vi "Send Example.vi"(0 "Input Data":T1 {"Command" format="%02x"; "Destination" format="%02x"; "Source" format="%02x"}, 1 "Retry Count":u8=5, 5 "Timeout (ms)":u32=500, 7 "Wait for Acknowledgement?":bool, 11 "Error In":errorcluster) -> (15 "Error Out":errorcluster)   [LabVIEW 2016]
doc: "This standalone VI sends a GEA2 message to the destination you specify."
uses:
  LabVIEW_GEA2_Toolkit.lvlibp/type defs/Data In.ctl
  LabVIEW_GEA2_Toolkit.lvlibp
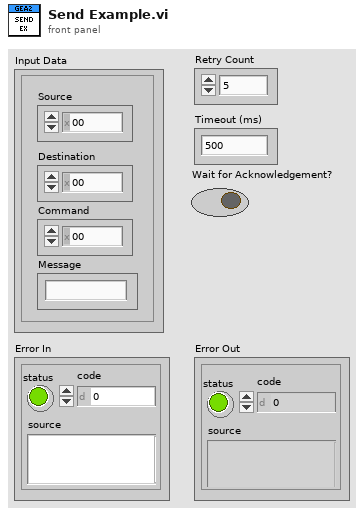
[diagram p1: front panel]
types:
  T1 = typedef "LabVIEW_GEA2_Toolkit.lvlibp/Data In.ctl" = cluster{"Source":u8, "Destination":u8, "Command":u8, "Message":string}
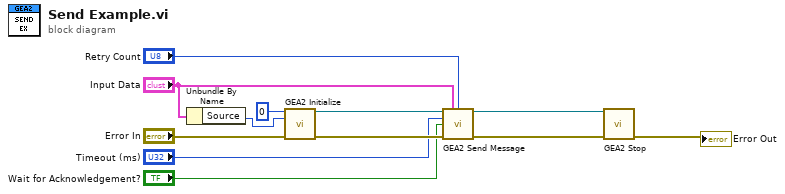
[diagram p0: block diagram]
diagram:
  n1 = Unbundle By Name("Input Data") -> ("Source"=w3:u8)
  n2 = call "GEA2 Initialize.vi"("Board Index"=0, "Source Address"=w3, "error in"="Error In") -> ("GEA2 Reference Out"=w12:refnum<k24>, "error out"=w9:errorcluster)  [unwired: 10 in, 1 out]
  n3 = call "GEA2 Send Message.vi"("GEA2 Reference In"=w12, "Input Data"="Input Data", "# of Tries"="Retry Count", "Timeout (ms)"="Timeout (ms)", "Wait for Acknowledgement?"="Wait for Acknowledgement?", "Error In"=w9) -> ("GEA2 Reference Out"=w11:refnum<k24>, "Error Out"=w10:errorcluster)  [unwired: 8 in]
  n4 = call "GEA2 Stop.vi"("GEA2 Reference In"=w11, "Error In"=w10) -> ("Error Out"=→"Error Out":errorcluster)  [unwired: 13 in]
